vi "saturateCtrlEff.vi"(9 "Upper Limit (10)":fxp<+/-,25,5>[](array[numeric])=[10.0, 10.0, 10.0, 10.0, 10.0], 10 "Lower Limit (-10)":fxp<+/-,25,5>[](array[numeric])=[-10.0, -10.0, -10.0, -10.0, -10.0], 11 "Array In":fxp<+/-,25,5>[](array[numeric])=[0.0, 0.0, 0.0, 0.0, 0.0]) -> (3 "Array Out":fxp<+/-,25,5>[](array[numeric]))   [LabVIEW 2020, in "CtrlEff.lvlib"]
doc: "Saturates the control efforts based on upper and lower limits."
uses:
  CtrlEff.lvlib
  <vilib>/Platform/TimedLoop/XDataNode/timing_clust.ctl
  <vilib>/Platform/TimedLoop/XDataNode/nitl_modes.ctl
  <vilib>/Platform/TimedLoop/XDataNode/wakeup.ctl
  <vilib>/rvi/Emulation/niFpgaSctlEmulationGetInTimedLoop.vi
  <vilib>/rvi/Emulation/niFpgaEmulationReportErrorSimple.vi
  <vilib>/rvi/Emulation/niFpgaGetClockAttributes.vi
  <vilib>/rvi/Emulation/niFpgaCriticalErrorInLSC.vi
  <vilib>/Platform/TimedLoop/XDataNode/XDataNode.xnode
  <vilib>/Platform/TimedLoop/XDataNode/XDNodeRunTimeDep.lvlib
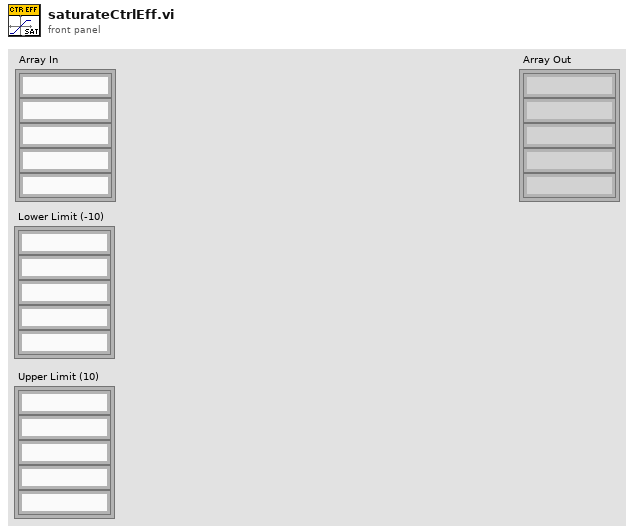
[diagram p1: front panel]
types:
  T1 = typedef "XDNodeRunTimeDep.lvlib/timing_clust.ctl" = cluster{"Expected End [f-1]":u64, "Actual End [f-1]":u64, "Finished Late? [f-1]":bool, "Expected End [i-1]":u64, "Actual End [i-1]":u64, "Finished Late? [i-1]":bool, "Expected Start [i]":u64, "Actual Start [i]":u64, "Expected Start [f]":u64, "Actual Start [f]":u64, "Source Name":string, "Structure Name":string, "Period":i64, "Deadline":i64, "Offset":i64, "Start":i64, "Priority":i32, "Timeout":i32, "Mode":T2, "Wakeup Reason":T3, "Error":errorcluster, "Source Type":string, "Secondary Source Type":string, "Global End Time":u64, "Global Start Time":u64, "Frame Duration":u64, "Iteration Duration":u64, "Assigned CPU":i32, "I/O Scan Engine Mode":u32}
  T2 = typedef "XDNodeRunTimeDep.lvlib/nitl_modes.ctl" = enum32{"No Change", "Process missed periods, maintain original phase", "Discard missed periods, maintain original phase", "Process missed periods, ignore original phase", "Discard missed periods, ignore original phase"}
  T3 = typedef "XDNodeRunTimeDep.lvlib/wakeup.ctl" = enum32{"Normal", "Aborted", "Asynchronous wakeup", "Timing source error", "Timed loop error", "Timeout"}
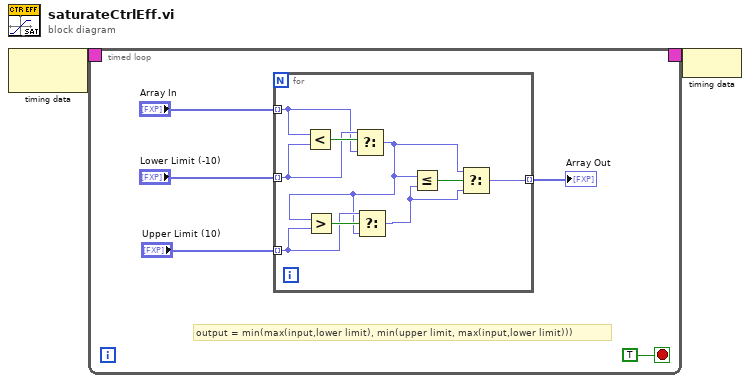
[diagram p0: block diagram]
diagram:
  n1 = node-c288() -> (w2:T1)  [unwired: 1 in]
  n2 = timed-loop {
    timing: w2 -> [_]
    timing-out: [_] -> w1
    stop <- TRUE stop-if-true
    # "output = min(max(input,lower limit), min(upper limit, max(input,lower limit)))"
    n3 = for {
      tunnel: "Array In" -> [w12] mode=indexing
      tunnel: "Lower Limit (-10)" -> [w13] mode=indexing
      tunnel: "Upper Limit (10)" -> [w15] mode=indexing
      tunnel: [w9] -> w4 mode=indexing
      n4 = Less?(x=w12, y=w13) -> (x < y?=w14:bool)
      n5 = Select(t=w13, s=w14, f=w12) -> (s? t:f=w8:fxp<+/-,25,5>)
      n6 = Greater?(x=w8, y=w15) -> (0:w16:bool)
      n7 = Select(t=w15, s=w16, f=w8) -> (s? t:f=w10:fxp<+/-,25,5>)
      n8 = Less Or Equal?(x=w8, y=w10) -> (x <= y?=w11:bool)
      n9 = Select(t=w8, s=w11, f=w10) -> (s? t:f=w9:fxp<+/-,25,5>)
    }
    "Array Out" <- w4
  }
  n10 = node-c288(w1) -> ()
